vi "robot_stay.vi"(5 "Vz":dbl, 6 "Z":dbl, 7 "Vy":dbl, 8 "Y":dbl, 9 "X":dbl, 10 "Active?":bool[](array[boolean])=[TRUE, TRUE, TRUE], 11 "Vx":dbl) -> (0 "Fz":dbl, 1 "Fy":dbl, 2 "Fx":dbl)   [LabVIEW 2012]
uses:
  Global_var.vi
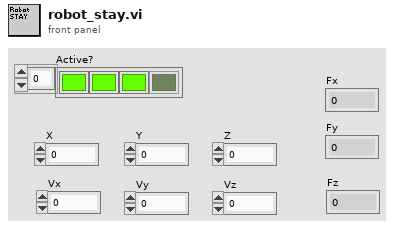
[diagram p1: front panel]
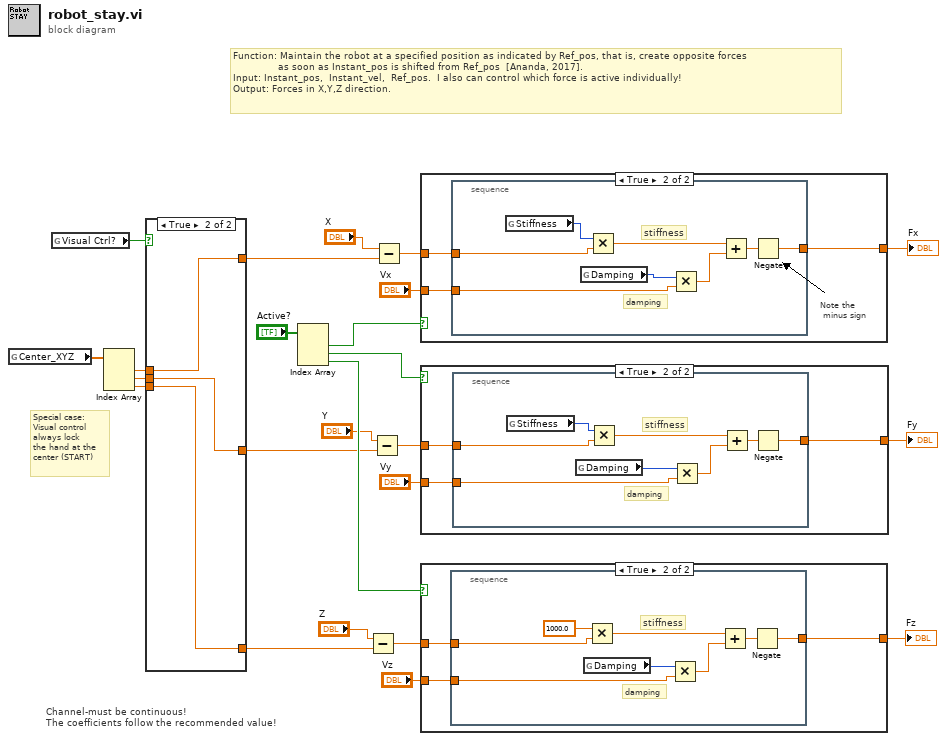
[diagram p0: block diagram]
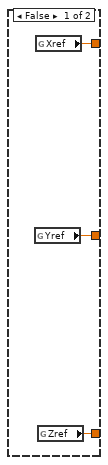
[diagram p2: hidden frame]
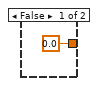
[diagram p3: hidden frame]
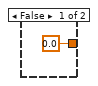
[diagram p4: hidden frame]
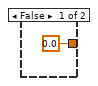
[diagram p5: hidden frame]
diagram:
  # "Special case:\nVisual control\nalways lock\nthe hand at the\ncenter (START)"
  # "Channel-must be continuous! \nThe coefficients follow the recommended value!"
  # "Function: Maintain the robot at a specified position as indicated by Ref_pos, that is, create opposite forces \n               as soon as Instant_pos is shifted from Ref_pos  [Ananda, 2017].\nInput: Instant_pos,  Instant_vel,  Ref_pos.  I also can control which force is active individually!\nOutput: Forces in X,Y,Z direction."
  n1 = global read "Global_var.vi" "Center_XYZ"() -> (w4:dbl[])
  n2 = global read "Global_var.vi" "Visual Ctrl?"() -> (w5:bool)
  n3 = Index Array(array=w4) -> (element #1=w3:dbl, element #2=w2:dbl, element #3=w1:dbl)  [unwired: 3 in]
  n4 = case shown="True" w5 {
    tunnel: [w27 w30] -> w16
    tunnel: [w26 w29] -> w11
    tunnel: [w25 w28] -> w8
    tunnel: w3 -> [_ w30]
    tunnel: w2 -> [_ w29]
    tunnel: w1 -> [_ w28]
    frame False {
      n5 = global read "Global_var.vi" "Yref"() -> (w26:dbl)
      n6 = global read "Global_var.vi" "Xref"() -> (w27:dbl)
      n7 = global read "Global_var.vi" "Zref"() -> (w25:dbl)
    }
    frame True {
    }
  }
  n8 = Index Array(array="Active?") -> (element #1=w21:bool, element #2=w20:bool, element #3=w19:bool)  [unwired: 3 in]
  n9 = Subtract(x="Z", y=w8) -> (x-y=w7:dbl)
  n10 = Subtract(x="Y", y=w11) -> (x-y=w10:dbl)
  n11 = Subtract(x="X", y=w16) -> (x-y=w15:dbl)
  n12 = case shown="True" w21 {
    tunnel: [0.0 w34] -> w24
    tunnel: w15 -> [_ w33]
    tunnel: "Vx" -> [_ w32]
    frame False {
    }
    frame True {
      # "Note the\n minus sign"
      n13 = stacked-sequence {
        tunnel: [w37] -> w34
        tunnel: w33 -> [w38]
        tunnel: w32 -> [w39]
        frame #0 {
          # "stiffness"
          # "damping"
          n14 = global read "Global_var.vi" "Stiffness"() -> (w35:i16)
          n15 = global read "Global_var.vi" "Damping"() -> (w36:i16)
          n16 = Multiply(x=w35, y=w38) -> (x*y=w41:dbl)
          n17 = Multiply(x=w36, y=w39) -> (x*y=w42:dbl)
          n18 = Add(x=w41, y=w42) -> (x+y=w40:dbl)
          n19 = Negate(x=w40) -> (-x=w37:dbl)
        }
      }
    }
  }
  "Fx" <- w24
  n20 = case shown="True" w20 {
    tunnel: "Vy" -> [_ w46]
    tunnel: [0.0 w45] -> w23
    tunnel: w10 -> [_ w44]
    frame False {
    }
    frame True {
      n21 = stacked-sequence {
        tunnel: [w50] -> w45
        tunnel: w46 -> [w51]
        tunnel: w44 -> [w47]
        frame #0 {
          # "stiffness"
          # "damping"
          n22 = global read "Global_var.vi" "Stiffness"() -> (w48:i16)
          n23 = global read "Global_var.vi" "Damping"() -> (w49:i16)
          n24 = Multiply(x=w48, y=w47) -> (x*y=w53:dbl)
          n25 = Multiply(x=w49, y=w51) -> (x*y=w54:dbl)
          n26 = Add(x=w53, y=w54) -> (x+y=w52:dbl)
          n27 = Negate(x=w52) -> (-x=w50:dbl)
        }
      }
    }
  }
  "Fy" <- w23
  n28 = case shown="True" w19 {
    tunnel: [0.0 w58] -> w22
    tunnel: w7 -> [_ w57]
    tunnel: "Vz" -> [_ w56]
    frame False {
    }
    frame True {
      n29 = stacked-sequence {
        tunnel: [w61] -> w58
        tunnel: w57 -> [w62]
        tunnel: w56 -> [w63]
        frame #0 {
          # "stiffness"
          # "damping"
          n30 = global read "Global_var.vi" "Damping"() -> (w60:i16)
          n31 = Multiply(x=1000.0, y=w62) -> (x*y=w65:dbl)
          n32 = Multiply(x=w60, y=w63) -> (x*y=w66:dbl)
          n33 = Add(x=w65, y=w66) -> (x+y=w64:dbl)
          n34 = Negate(x=w64) -> (-x=w61:dbl)
        }
      }
    }
  }
  "Fz" <- w22
